vi "Time (Read).vi"(6 "ISOBUS address":T2=-1 caption="ISOBUS address (-1)", 8 "error in":errorcluster, 11 "Mercury Reference In":T3) -> (0 "error out":errorcluster, 2 "Time":string, 3 "Mercury Reference Out":T3, 4 "Valid?":T1)   [LabVIEW 2014, in "Mercury iXX.lvlib" / "System.lvlib"]
doc: "Returns the current time according to the instrument."
uses:
  System.lvlib
  Controls/Mercury Reference.ctl
  Controls/Comms Transport Layer.ctl
  Private/Controls/Query Dynamic Reference.ctl
  Controls/ISOBus Address.ctl
  Controls/Is Valid LED.ctl
  Mercury iXX.lvlib
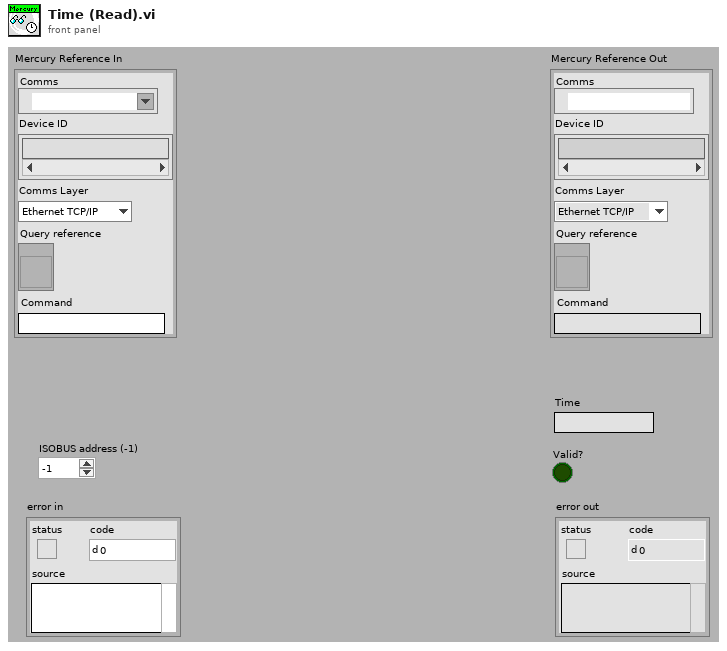
[diagram p1: front panel]
types:
  T1 = typedef "Mercury iXX.lvlib/Is Valid LED.ctl" = bool
  T2 = typedef "Mercury iXX.lvlib/ISOBus Address.ctl" = i32
  T3 = typedef "Mercury iXX.lvlib/Mercury Reference.ctl" = cluster{"Comms":refnum<visa-resource-name>, "Device ID":string[], "Comms Layer":T4, "Command":string, "Query reference":T5}
  T4 = typedef "Mercury iXX.lvlib/Comms Transport Layer.ctl" = enum16{"Ethernet TCP/IP", "USB", "ISOBus - RS-232", "GPIB"}
  T5 = typedef "Mercury iXX.lvlib/Query Dynamic Reference.ctl" = refnum<vi>
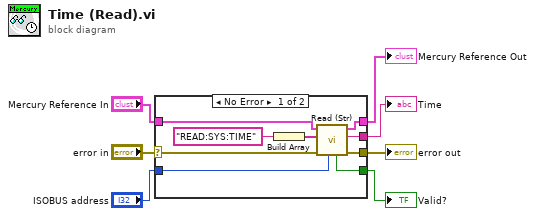
[diagram p0: block diagram]
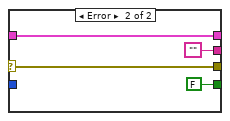
[diagram p2: hidden frame]
diagram:
  n1 = case shown="No Error" "error in" {
    selector: "error in" -> [w10 w19]
    tunnel: "Mercury Reference In" -> [w16 w20]
    tunnel: [w15 w20] -> w6
    tunnel: [w11 w19] -> w5
    tunnel: "ISOBUS address" -> [w14 _]
    tunnel: [w12 ""] -> w2
    tunnel: [w13 FALSE ("Valid?")] -> w1
    frame No Error {
      n2 = Build Array("READ:SYS:TIME" ("Command")) -> (w8:string[])
      n3 = call "Read (Str).vi"("ISOBUS address"=w14, "error in"=w10, "SCPI Message(s)"=w8, "Mercury Reference In"=w16) -> ("error out"=w11:errorcluster, "Response"=w12:string, "Mercury Reference Out"=w15:T3, "Valid?"=w13:T1)  [unwired: 4 out]
    }
    frame Error {
    }
  }
  "Mercury Reference Out" <- w6
  "error out" <- w5
  "Time" <- w2
  "Valid?" <- w1
